vi "Sample_Scan_Picture.vi"() -> ()   [LabVIEW 2013]
panel:
  in  "pen":T1={"Width"=1, "Style"=enum."Solid"}
  out "new picture":picture
  in  "line endpoints":cluster{"x":i16, "y":i16}[](array[cluster])
  in  "picture":picture
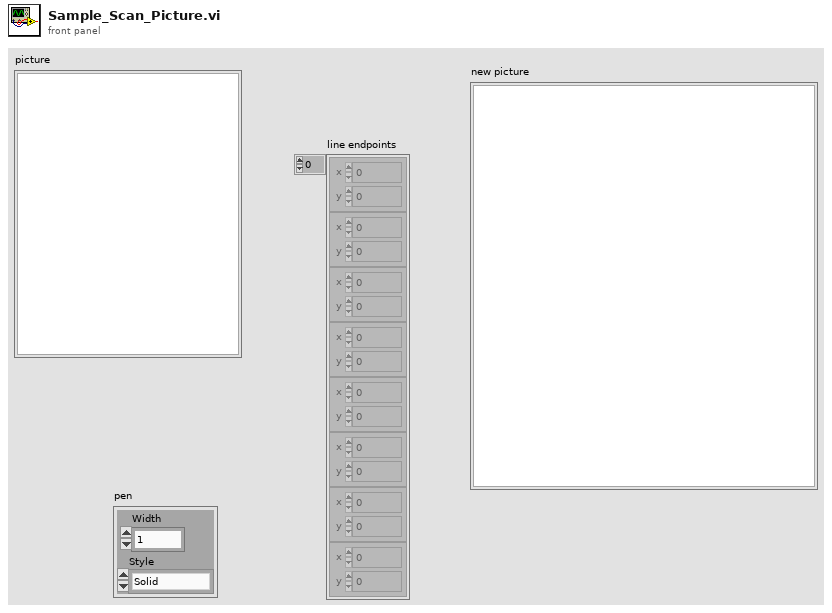
[diagram p1: front panel]
types:
  T1 = cluster{"Width":u16, "Style":enum32{"Solid", "Dash", "Dot", "DashDot", "DashDotDot"}}
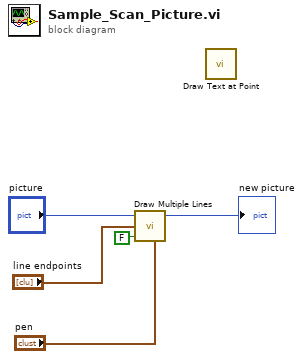
[diagram p0: block diagram]
diagram:
  n1 = call <vilib>:"Draw Multiple Lines.vi"("picture"="picture", "line endpoints"="line endpoints", "fill?(F)"=FALSE, "pen"="pen") -> ("new picture"=→"new picture":picture)  [unwired: 5 in]
  n2 = call <vilib>:"Draw Text at Point.vi"() -> ()  [unwired: 10 in, 2 out]
